vi "Get INI Section.vi"(4 "error IN":errorcluster, 5 "Ring Refnum":refnum<vi>, 6 "Sort":bool, 7 "configuration file path":path) -> (0 "error OUT":errorcluster, 3 "Array":string[](array[string]))   [LabVIEW 2015]
uses:
  <vilib>/Utility/config.llb/Read Key (String).vi
  <vilib>/Utility/config.llb/NI_LVConfig.lvlib
panel:
  out "section":string="Manufacturer"
  # "Sorted"
  # "Unsorted"
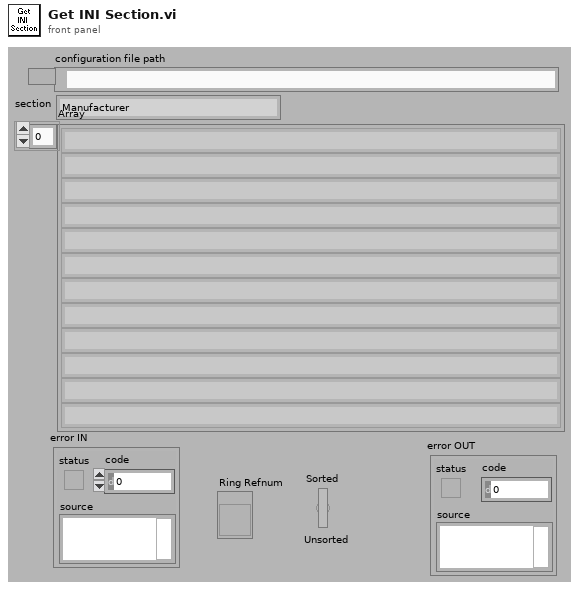
[diagram p1: front panel]
types:
  T1 = typedef "NI_LVConfig.lvlib/Config Data RefNum.ctl" = refnum<k1>
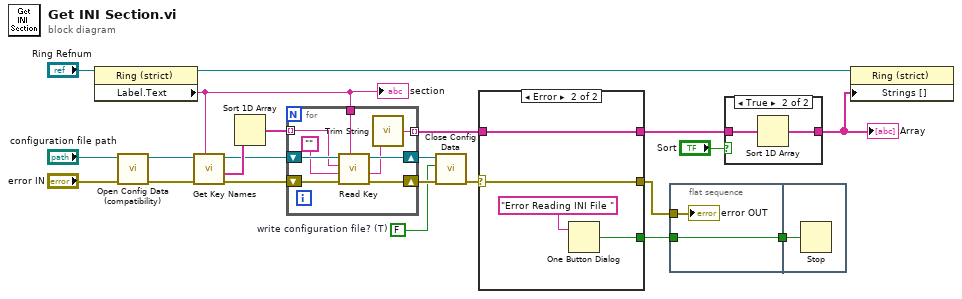
[diagram p0: block diagram]
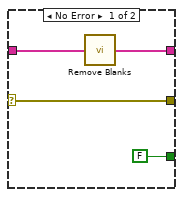
[diagram p3: hidden frame]
diagram:
  w8 = FALSE  # write configuration file? (T)
  n1 = property class="Ring (strict)"(reference="Ring Refnum") -> (reference out=w6:refnum<vi>, "Label.Text"=w4:string)  [unwired: 1 in, 1 out]
  "section" <- w4
  n2 = call <vilib>:"Open Config Data (compatibility).vi"("error in (no error)"="error IN", "configuration file path"="configuration file path") -> ("error out"=w16:errorcluster, "refnum"=w17:T1)  [unwired: 7 in, 1 out]
  n3 = call <vilib>:"Get Key Names.vi"("section"=w4, "error in (no error)"=w16, "refnum"=w17) -> ("error out"=w21:errorcluster, "key names"=w19:string[], "refnum out"=w18:T1)  [unwired: 6 out]
  n4 = Sort 1D Array(array=w19) -> (sorted array=w9:string[])
  n5 = for {
    tunnel: w9 -> [w29] mode=indexing
    tunnel: w4 -> [w26]
    tunnel: [w23] -> w12 mode=indexing
    shift-right: [w24] -> w15
    shift-left: w21 -> [w28]
    shift-right: [w30] -> w20
    shift-left: w18 -> [w31]
    n6 = call-poly <vilib>:"Read Key.vi"("section"=w26, "error in (no error)"=w28, "default value"="", "key"=w29, "refnum"=w31) -> ("error out"=w24:errorcluster, "value"=w25:string, "refnum out"=w30:T1)  [unwired: 1 in, 3 out]
    n7 = call "Trim String.vi"("inStr"=w25) -> ("outStr"=w23:string)
  }
  n8 = call <vilib>:"Close Config Data.vi"("error in (no error)"=w15, "write file if changed (T)"=w8, "refnum"=w20) -> ("error out"=w14:errorcluster)  [unwired: 8 out]
  n9 = case shown="Error" w14 {
    selector: w14 -> [w33 w37]
    tunnel: w12 -> [w35 w38]
    tunnel: [w34 w38] -> w10
    tunnel: [w33 w37] -> w3
    tunnel: [FALSE ("true") w36] -> w2
    frame No Error {
      n10 = call "Remove Blanks.vi"("INPUT STRING ARRAY"=w35) -> ("OUTPUT STRING ARRAY"=w34:string[])
    }
    frame Error {
      n11 = One Button Dialog(message="Error Reading INI File ") -> (true=w36:bool)  [unwired: 1 out]
    }
  }
  n12 = flat-sequence {
    tunnel: w3 -> [w41]
    tunnel: w2 -> [w40]
    tunnel: [w40] -> w1
    tunnel: w1 -> [w42]
    frame #0 {
      "error OUT" <- w41
    }
    frame #1 {
      n13 = Stop(stop? (T)=w42) -> ()
    }
  }
  n14 = case shown="True" "Sort" {
    tunnel: w10 -> [w43 w45]
    tunnel: [w43 w44] -> w5
    frame False {
    }
    frame True {
      n15 = Sort 1D Array(array=w45) -> (sorted array=w44:string[])
    }
  }
  "Array" <- w5
  n16 = property class="Ring (strict)"(reference=w6, "Strings []"=w5) -> ()  [unwired: 1 in, 2 out]
